vi "Write FIFO (Two Channels).vi"(0 "data in":u32[](array[numeric]), 1 "fifo 0":refnum<k21>, 2 "fifo 1":refnum<k21>, 5 "enable":bool[](array[boolean]), 9 "input valid":bool) -> (14 "ready for input":bool)   [LabVIEW 2018]
doc: "Writes data to two 32-bit FIFOs. This VI is a wrapper around the LabVIEW FPGA FIFO Write method. This VI exposes handshaking signals that inform the user when the FIFOs are ready to accept new data.\n\n<B>Input Parameters</B>\n\n<B>data in</B> is the data to be written to the FIFO.\n\n<B>enabled</B> specifies which streams are enabled.\n\n<B>input valid</B> specifies when 'data in' is valid.\n\n<B>reset</B> the LabVIEW FPGA FIFO.\n\n<B>fifo 0</B> is the reference to the FIFO to which data received on channel 0 will be written to.\n\n<B>fifo 1</B> is the reference to the FIFO to which data received on channel 1 will be written to.\n\n<B>Output Parameters</B>\n\n<B>ready for input</B> is a flow control signal that indicates whether the Write FIFO VI is ready to accept new data."
uses:
  <vilib>/rvi/DataTransferAndStorage/Container/Common/niFpgaContainerExecOnDevCompGetState.vi
  <vilib>/rvi/Emulation/niFpgaEmulationIsFPGAContextNoSignature.vi
  <vilib>/rvi/Emulation/niFpgaSctlEmulationGetInTimedLoop.vi
  <vilib>/rvi/errors/niFpgaSetErrorForExecOnDevCompSimple.vi
  <vilib>/rvi/eio/common/nirviEmuReportErrorAndStop.vi
  <vilib>/rvi/DataTransferAndStorage/Container/Common/niFpgaContainerGetUniqueNameForEmu.vi
  <vilib>/rvi/FIFO/Fifo_Resource/nirvififoEmulationSetSize.vi
  <vilib>/rvi/FIFO/Fifo_Resource/nirviFifoEmulationQueueMgr.vi
  <instcachedir>/0/nirviFifoEmulationQueueMgr_E5CAEC123FF24DC58D834DCA3CDAA9B5.lvgen/nirviFifoEmulationQueueMgr_E5CAEC123FF24DC58D834DCA3CDAA9B5_001.vi
  <vilib>/rvi/FIFO/Fifo_Resource/nirvififoEmulationDetermineInputValidOut.vi
  <vilib>/rvi/FIFO/Fifo_Resource/nirvififoEmulationCreateLock.vi
  <vilib>/rvi/Emulation/niFpgaProcessEmulError.vi
  <vilib>/rvi/FIFO/Fifo_Resource/nirvififoEmulationObtainLock.vi
  <vilib>/rvi/FIFO/Fifo_Resource/nirvififoEmulationReleaseLock.vi
  <vilib>/rvi/occurrence/nirviWaitOnOccurrenceBase.vi
  <vilib>/rvi/errors/nirviReportUnexpectedCaseInternalError.vi
  <vilib>/rvi/errors/nirviReportUnexpectedCaseInternalError (U32).vi
  <vilib>/Utility/error.llb/Clear Errors.vi
  <vilib>/rvi/interface/RandomDataEmulation/niFpgaRandomDataHandleErrors.vi
  <vilib>/rvi/DataTransferAndStorage/Container/XNode/niFpgaContainer.xnode
  <vilib>/rvi/FIFO/Fifo_Resource/niFpgaFifoEmulationRefIn.vi
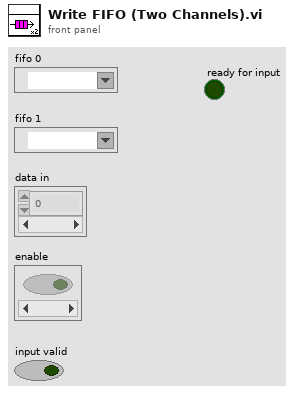
[diagram p1: front panel]
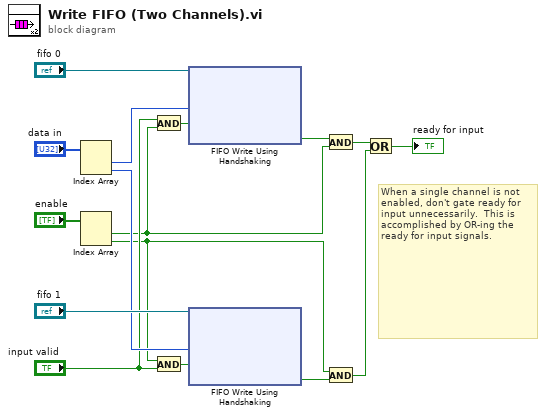
[diagram p0: block diagram]
diagram:
  # "When a single channel is not enabled, don't gate ready for input unnecessarily.  This is accomplished by OR-ing the ready for input signals."
  n1 = Index Array(array="data in") -> (element #1=w10:u32, element #2=w8:u32)  [unwired: 2 in]
  n2 = Index Array(array="enable") -> (element #1=w6:bool, element #2=w1:bool)  [unwired: 2 in]
  n3 = And(x="input valid", y=w6) -> (x .and. y?=w12:bool)
  n4 = And(x=w1, y="input valid") -> (x .and. y?=w9:bool)
  n5 = xnode "FIFO Write Using Handshaking"("要素"=w10, "入力有効"=w12, "FIFO入力"="fifo 0") -> ("入力準備完了"=w11:bool)  [unwired: 1 out]
  n6 = xnode "FIFO Write Using Handshaking"("要素"=w8, "入力有効"=w9, "FIFO入力"="fifo 1") -> ("入力準備完了"=w2:bool)  [unwired: 1 out]
  n7 = And(x=w11, y=w6) -> (x .and. y?=w5:bool)
  n8 = And(x=w1, y=w2) -> (x .and. y?=w4:bool)
  n9 = Or(x=w5, y=w4) -> (x .or. y?=→"ready for input":bool)
